vi "ADAM Get Relay States.vi"() -> ()   [LabVIEW 2018]
uses:
  nimodbus121/71/vi.lib/NI Modbus.llb/MB Modbus Command.ctl
panel:
  out "error out":errorcluster
  in  "Modbus Command":T1={"Function Code"=3, "Starting Address"=0, "Quantity"=1, "Data"=[], "Discrete"=[]} {"Function Code" items=["Read Coils"=1, "Read Discrete Inputs"=2, "Read Holding Registers"=3, "Read Input Registers"=4, "Write Single Coil"=5, "Write Single Register"=6, "Read Exception Status"=7, "Write Multiple Coils"=15, "Write Multiple Registers"=16]}
  in  "stop":bool
  out "Slave Input Registers 2":u16[](array[numeric]) caption="Slave Input Registers (Read Only)"
  in  "Remote Port 2":u16=502
  in  "Remote IP Address 2":string="192.168.10.200"
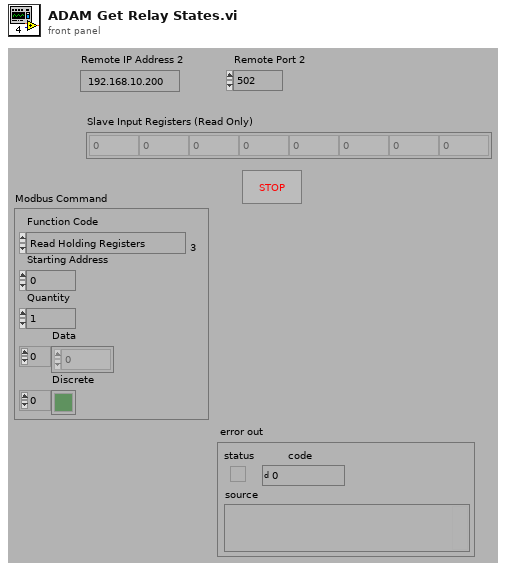
[diagram p1: front panel]
types:
  T1 = typedef "MB Modbus Command.ctl" = cluster{"Function Code":u8, "Starting Address":u16, "Quantity":u16, "Data":u16[], "Discrete":bool[]}
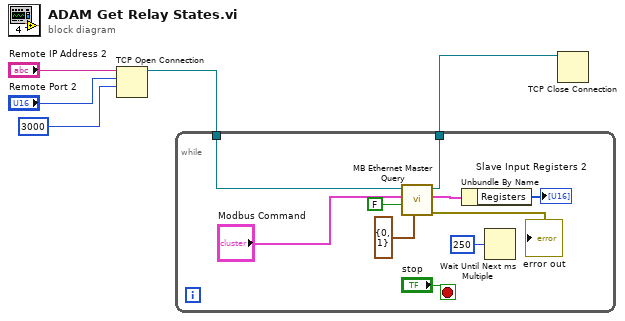
[diagram p0: block diagram]
diagram:
  n1 = TCP Open Connection(address="Remote IP Address 2", remote port or service name="Remote Port 2", timeout ms (60000)=3000) -> (connection ID=w3:refnum<k5>)  [unwired: 2 in, 1 out]
  n2 = while {
    tunnel: w3 -> [w12]
    tunnel: [w11] -> w2
    stop <- "stop" stop-if-true
    n3 = call "MB Ethernet Master Query.vi"("MBAP Header"=cluster{"Transaction ID":u16, "Unit ID":u8} {"Transaction ID"=0, "Unit ID"=1}, "Use MODBUS Data Unit?"=FALSE, "Modbus Command"="Modbus Command", "TCP Connection Refnum in"=w12) -> ("error out"=→"error out":errorcluster, "Registers"=w13:cluster{"Registers":u16[], "Discrete":bool[]}, "TCP Connection Refnum (dup)"=w11:refnum<k5>)  [unwired: 3 in, 2 out]
    n4 = Unbundle By Name(w13) -> ("Registers"=→"Slave Input Registers 2":u16[])
    n5 = Wait Until Next ms Multiple(millisecond multiple=u32 250) -> ()  [unwired: 1 out]
  }
  n6 = TCP Close Connection(connection ID=w2) -> ()  [unwired: 2 in, 2 out]
